vi "Terminal_PerssureSyetem_Work_Condition.vi"(11 "液压子系统监测参数":T1) -> (3 "达到工作条件":bool)   [LabVIEW 2014]
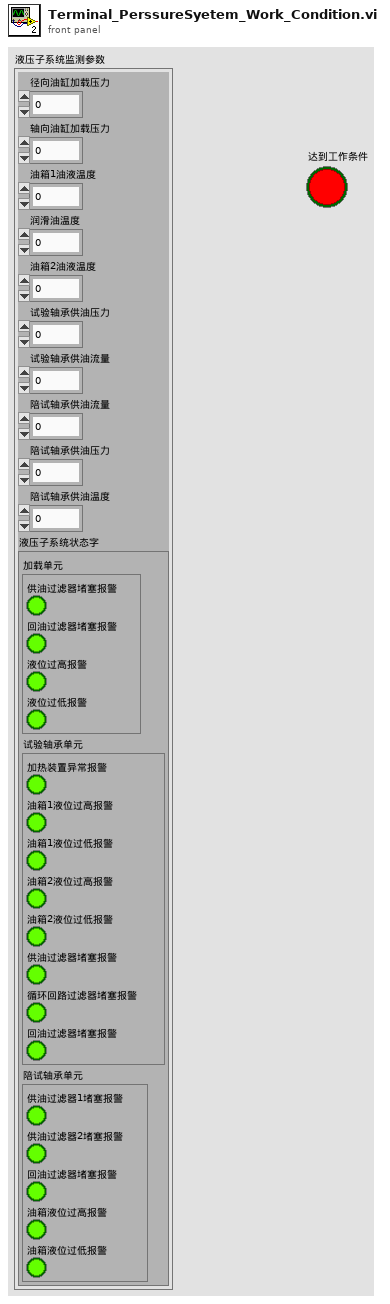
[diagram p1: front panel]
types:
  T1 = cluster{"径向油缸加载压力":u16, "轴向油缸加载压力":u16, "油箱1油液温度":u16, "润滑油温度":u16, "油箱2油液温度":u16, "试验轴承供油压力":u16, "试验轴承供油流量":u16, "陪试轴承供油流量":u16, "陪试轴承供油压力":u16, "陪试轴承供油温度":u16, "液压子系统状态字":cluster{"加载单元":cluster{"供油过滤器堵塞报警":bool, "回油过滤器堵塞报警":bool, "液位过高报警":bool, "液位过低报警":bool}, "试验轴承单元":cluster{"加热装置异常报警":bool, "油箱1液位过高报警":bool, "油箱1液位过低报警":bool, "油箱2液位过高报警":bool, "油箱2液位过低报警":bool, "供油过滤器堵塞报警":bool, "循环回路过滤器堵塞报警":bool, "回油过滤器堵塞报警":bool}, "陪试轴承单元":cluster{"供油过滤器1堵塞报警":bool, "供油过滤器2堵塞报警":bool, "回油过滤器堵塞报警":bool, "油箱液位过高报警":bool, "油箱液位过低报警":bool}}}
  T2 = cluster{"加载单元":cluster{"供油过滤器堵塞报警":bool, "回油过滤器堵塞报警":bool, "液位过高报警":bool, "液位过低报警":bool}, "试验轴承单元":cluster{"加热装置异常报警":bool, "油箱1液位过高报警":bool, "油箱1液位过低报警":bool, "油箱2液位过高报警":bool, "油箱2液位过低报警":bool, "供油过滤器堵塞报警":bool, "循环回路过滤器堵塞报警":bool, "回油过滤器堵塞报警":bool}, "陪试轴承单元":cluster{"供油过滤器1堵塞报警":bool, "供油过滤器2堵塞报警":bool, "回油过滤器堵塞报警":bool, "油箱液位过高报警":bool, "油箱液位过低报警":bool}}
  T3 = cluster{"供油过滤器堵塞报警":bool, "回油过滤器堵塞报警":bool, "液位过高报警":bool, "液位过低报警":bool}
  T4 = cluster{"加热装置异常报警":bool, "油箱1液位过高报警":bool, "油箱1液位过低报警":bool, "油箱2液位过高报警":bool, "油箱2液位过低报警":bool, "供油过滤器堵塞报警":bool, "循环回路过滤器堵塞报警":bool, "回油过滤器堵塞报警":bool}
  T5 = cluster{"供油过滤器1堵塞报警":bool, "供油过滤器2堵塞报警":bool, "回油过滤器堵塞报警":bool, "油箱液位过高报警":bool, "油箱液位过低报警":bool}
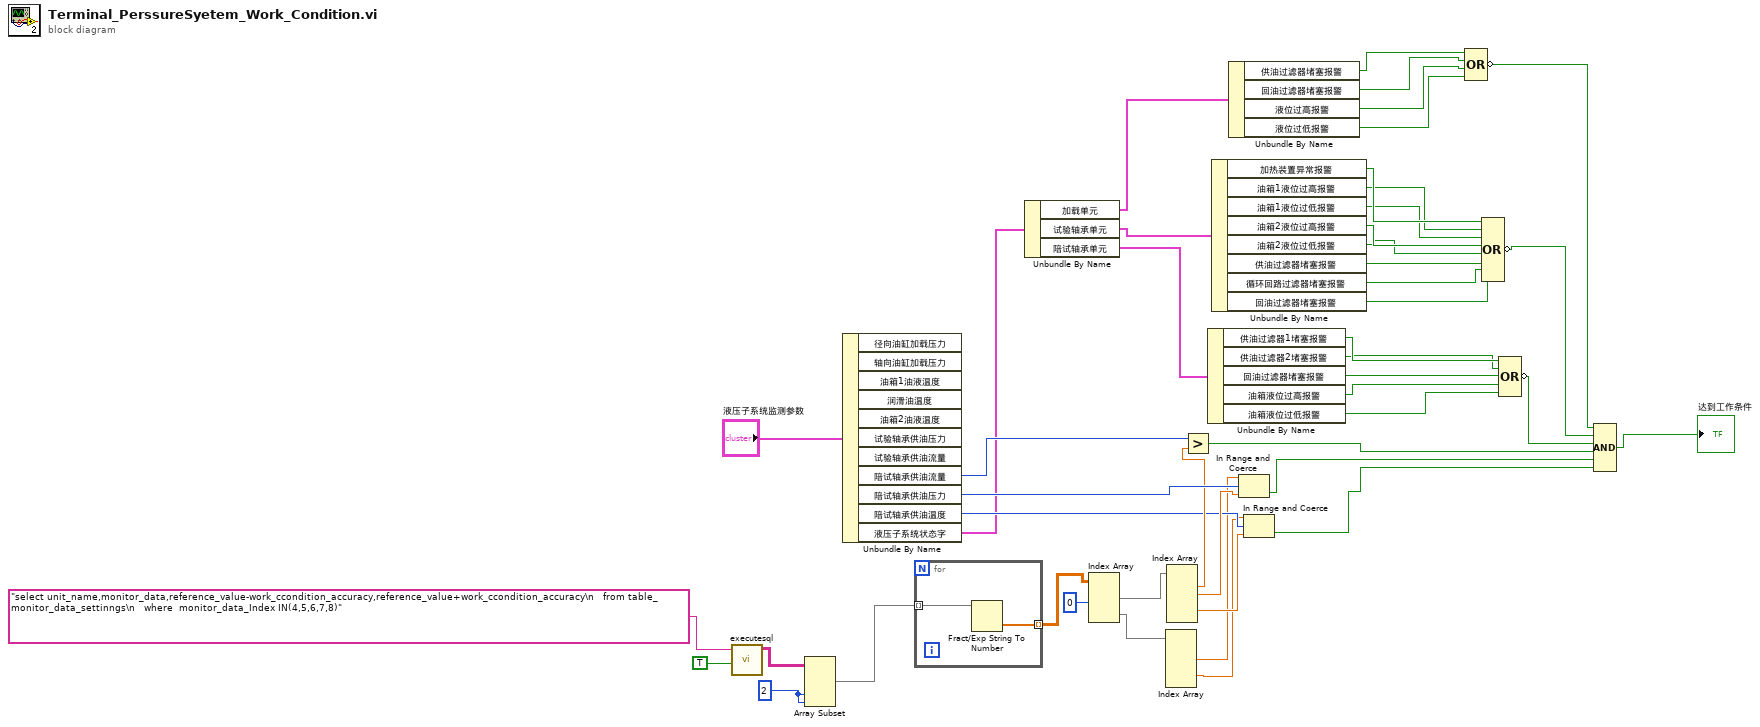
[diagram p0: block diagram]
diagram:
  w43 = 2
  n1 = call "executesql.vi"("Return Data (T)"=TRUE, "Command Text"="select unit_name,monitor_data,reference_value-work_ccondition_accuracy,reference_value+work_ccondition_accuracy\n   from table_monitor_data_settinngs\n   where  monitor_data_Index IN(4,5,6,7,8)") -> ("Data"=w44:string[][])  [unwired: 5 in, 1 out]
  n2 = Array Subset(array=w44, index (col)=w43, length (col)=w43) -> (w40:string[][])  [unwired: 2 in]
  n3 = Unbundle By Name("液压子系统监测参数") -> ("陪试轴承供油流量"=w41:u16, "陪试轴承供油压力"=w39:u16, "陪试轴承供油温度"=w33:u16, "液压子系统状态字"=w25:T2)  [unwired: 7 out]
  n4 = for {
    tunnel: w40 -> [w48] mode=indexing
    tunnel: [w47] -> w38 mode=indexing
    n5 = Fract/Exp String To Number(string=w48) -> (number=w47:dbl[])  [unwired: 3 in, 1 out]
  }
  n6 = Unbundle By Name(w25) -> ("加载单元"=w24:T3, "试验轴承单元"=w23:T4, "陪试轴承单元"=w22:T5)
  n7 = Index Array(array=w38, index (col) #1=0) -> (element #1=w36:dbl[], element #2=w31:dbl[])  [unwired: 3 in]
  n8 = Index Array(array=w31) -> (element #2=w30:dbl, element #4=w29:dbl)  [unwired: 5 in, 3 out]
  n9 = Index Array(array=w36) -> (element #1=w35:dbl, element #2=w34:dbl, element #4=w32:dbl)  [unwired: 5 in, 2 out]
  n10 = Greater?(x=w41, y=w35) -> (0:w28:bool)
  n11 = Unbundle By Name(w22) -> ("供油过滤器1堵塞报警"=w9:bool, "供油过滤器2堵塞报警"=w8:bool, "回油过滤器堵塞报警"=w7:bool, "油箱液位过高报警"=w6:bool, "油箱液位过低报警"=w5:bool)
  n12 = Unbundle By Name(w23) -> ("加热装置异常报警"=w17:bool, "油箱1液位过高报警"=w16:bool, "油箱1液位过低报警"=w15:bool, "油箱2液位过高报警"=w14:bool, "油箱2液位过低报警"=w13:bool, "供油过滤器堵塞报警"=w12:bool, "循环回路过滤器堵塞报警"=w11:bool, "回油过滤器堵塞报警"=w10:bool)
  n13 = Unbundle By Name(w24) -> ("供油过滤器堵塞报警"=w21:bool, "回油过滤器堵塞报警"=w20:bool, "液位过高报警"=w19:bool, "液位过低报警"=w18:bool)
  n14 = In Range and Coerce(upper limit=w30, x=w39, lower limit=w34) -> (In Range?=w27:bool)  [unwired: 1 out]
  n15 = In Range and Coerce(upper limit=w29, x=w33, lower limit=w32) -> (In Range?=w26:bool)  [unwired: 1 out]
  n16 = Compound Arithmetic op=OR(w21, w20, w19, w18) -> (invert w4:bool)
  n17 = Compound Arithmetic op=OR(w17, w16, w15, w14, w13, w12, w11, w10) -> (invert w3:bool)
  n18 = Compound Arithmetic op=OR(w9, w8, w7, w6, w5) -> (invert w2:bool)
  n19 = Compound Arithmetic op=AND(w4, w3, w2, w28, w27, w26) -> (→"达到工作条件":bool)
